vi "Init_uc480.vi"(10 "mode":i32(ring)=128 items=["BGRA8Packed"=0, "BGR8Packed"=1, "BGR565Packed"=2, "BGR5Packed"=3, "Mono8"=6, "SensorRaw8"=11, "UYVYPacked"=12, "UYVYMonoPacked"=13, "UYVYBayerPacked"=14, "CBYCRYPacked"=23, "BGRY8Packed"=24, "BGR10Packed"=25, "Mono12"=26, "SensorRaw12"=27, "Mono16"=28, "SensorRaw16"=29, "BGR12Unpacked"=30, "BGRA12Unpacked"=31, "Jpeg"=32, "SensorRaw10"=33, "Mono10"=34, "BGR10Unpacked"=35, "RGBA8Packed"=128, "RGB8Packed"=129, "RGBY8Packed"=152, "RGB10Packed"=153, "RGB12Unpacked"=158, "RGBA12Unpacked"=159, "RGB10Unpacked"=163, "RGB8Planar"=8321, "PreferPackedSourceFormat"=16384], 11 "s32Cam":i32) -> (2 "SerialNumber":string, 3 ".NET Refnum out":refnum<k24>)   [LabVIEW 2019]
doc: "Init and low-level parameters of uc480/ThorCam DCx cameras."
uses:
  C:/Program Files/Thorlabs/Scientific Imaging/DCx Camera Support/Develop/DotNet/uc480DotNet.dll
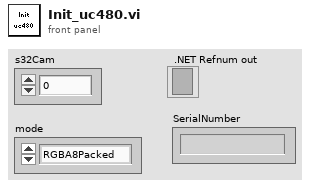
[diagram p1: front panel]
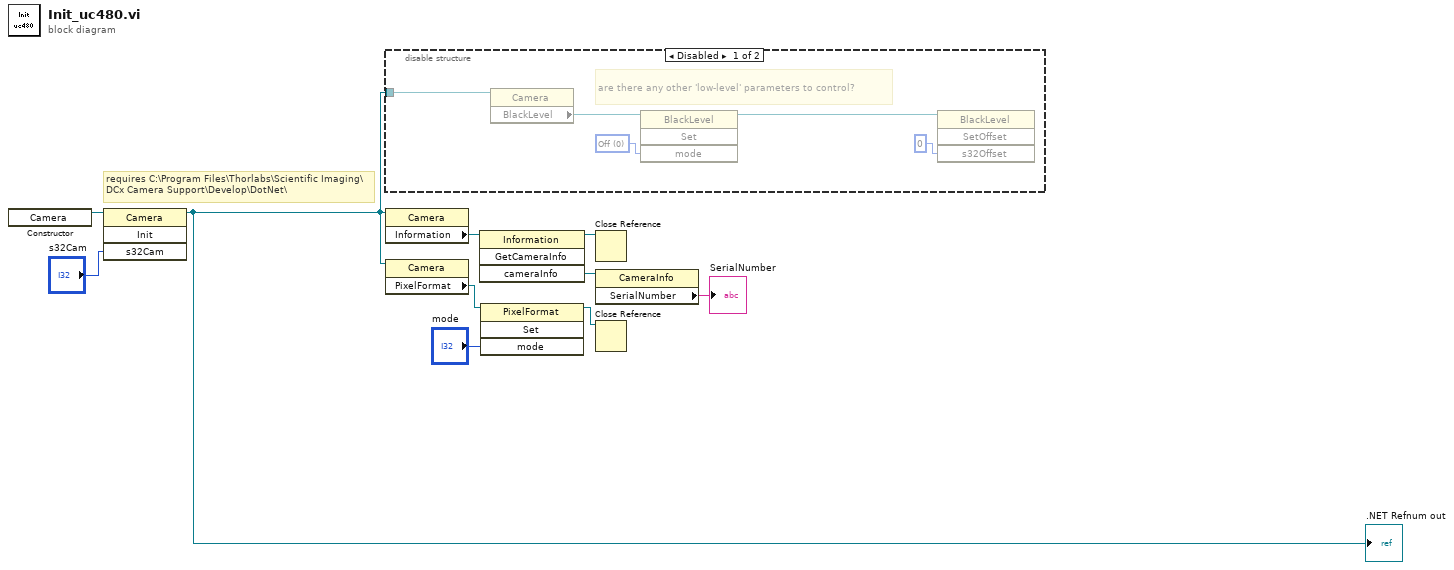
[diagram p0: block diagram]
diagram:
  # "requires C:\\Program Files\\Thorlabs\\Scientific Imaging\\DCx Camera Support\\Develop\\DotNet\\"
  n1 = constructor class="Camera"() -> (reference out=w9:refnum<k24>)  [unwired: 3 in, 2 out]
  n2 = invoke class="Camera" method="Init"(reference=w9, "s32Cam"="s32Cam") -> (reference out=w10:refnum<k24>)  [unwired: 2 in, 3 out]
  ".NET Refnum out" <- w10
  n3 = disable-structure shown="Disabled" {
    disable-tunnel: w10 -> [w11 _]
    frame Disabled {
      w15 = 0 items=["Off", "On"] ("mode")
      # "are there any other 'low-level' parameters to control?"
      n4 = property class="Camera"(reference=w11) -> ("BlackLevel"=w13:refnum<k24>)  [unwired: 1 in, 2 out]
      n5 = invoke class="BlackLevel" method="Set"(reference=w13, "mode"=w15) -> (reference out=w12:refnum<k24>)  [unwired: 2 in, 3 out]
      n6 = invoke class="BlackLevel" method="SetOffset"(reference=w12, "s32Offset"=0) -> ()  [unwired: 2 in, 4 out]
    }
    frame Enabled {
    }
  }
  n7 = property class="Camera"(reference=w10) -> ("Information"=w2:refnum<k24>)  [unwired: 1 in, 2 out]
  n8 = property class="Camera"(reference=w10) -> ("PixelFormat"=w6:refnum<k24>)  [unwired: 1 in, 2 out]
  n9 = invoke class="Information" method="GetCameraInfo"(reference=w2) -> (reference out=w5:refnum<k24>, "cameraInfo"=w3:refnum<k24>)  [unwired: 3 in, 2 out]
  n10 = invoke class="PixelFormat" method="Set"(reference=w6, "mode"="mode") -> (reference out=w8:refnum<k24>)  [unwired: 2 in, 3 out]
  n11 = Close Reference(reference=w5) -> ()  [unwired: 1 in, 1 out]
  n12 = property class="CameraInfo"(reference=w3) -> ("SerialNumber"=→"SerialNumber":string)  [unwired: 1 in, 2 out]
  n13 = Close Reference(reference=w8) -> ()  [unwired: 1 in, 1 out]
